vi "blue test 2.vi"   [LabVIEW 2010, in "Bluetooth.lvrbt"]
uses:
  Bluetooth.lvrbt
  <vilib>/NXT/Block Support/NXT_MessageMailbox.ctl
  <vilib>/NXT/Dual Mode Library/Display/drawNumber.vi
types:
  T1 = typedef "NXT_MessageMailbox.ctl" = u8
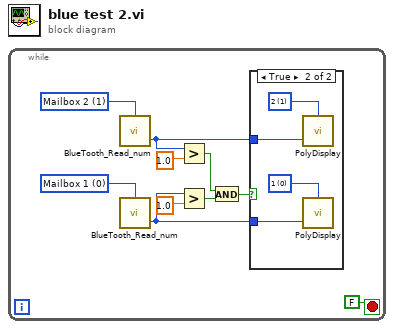
[diagram p0: block diagram]
diagram:
  n1 = while {
    stop <- FALSE stop-if-true
    w9 = T1 1 items=["Mailbox 1", "Mailbox 2", "Mailbox 3", "Mailbox 4", "Mailbox 5", "Mailbox 6", "Mailbox 7", "Mailbox 8", "Mailbox 9", "Mailbox 10"] ("Mailbox")
    w10 = T1 0 items=["Mailbox 1", "Mailbox 2", "Mailbox 3", "Mailbox 4", "Mailbox 5", "Mailbox 6", "Mailbox 7", "Mailbox 8", "Mailbox 9", "Mailbox 10"] ("Mailbox")
    n2 = call <vilib>:"BlueTooth_Read_num.vi"("Mailbox"=w9) -> ("Message"=w4:i32)  [unwired: 2 in, 1 out]
    n3 = call <vilib>:"BlueTooth_Read_num.vi"("Mailbox"=w10) -> ("Message"=w6:i32)  [unwired: 2 in, 1 out]
    n4 = Greater?(x=w4, y=1.0) -> (0:w3:bool)
    n5 = Greater?(x=w6, y=1.0) -> (0:w2:bool)
    n6 = And(x=w3, y=w2) -> (x .and. y?=w1:bool)
    n7 = case shown="True" w1 {
      tunnel: w6 -> [_ w12]
      tunnel: w4 -> [_ w11]
      frame False {
      }
      frame True {
        w13 = i16 1 items=["1", "2", "3", "4", "5", "6", "7", "8"] ("Line")
        w14 = i16 0 items=["1", "2", "3", "4", "5", "6", "7", "8"] ("Line")
        n8 = call-poly <vilib>:"PolyDisplay.vi"("number"=w11, "Line"=w13) -> ()  [unwired: 2 in, 1 out]
        n9 = call-poly <vilib>:"PolyDisplay.vi"("number"=w12, "Line"=w14) -> ()  [unwired: 2 in, 1 out]
      }
    }
  }
